vi "parse_variables.vi"(8 "error in (no error)":errorcluster, 9 "Cycles per Experiment":i32=1 min=1 step=1, 10 "Variables (Control)":string[][](table)=[["variable 1", "x", "500", "4000", "1"], ["variable 2", "y", "0", "0", "1"], ["variable 3", "z", "0", "0", "1"], ["", "", "", "", ""], ["", "", "", "", ""], ["", "", "", "", ""], ["", "", "", "", ""], ["", "", "", "", ""]] caption="(Inner loop at top)", 11 "base path":path) -> (0 "error out":errorcluster, 1 "variable indices":i32[][](array[numeric]), 2 "Step Sizes Array":dbl[](array[numeric]), 3 "Variable Names Array":string[](array[string]), 4 "Total Number of Data Points":i32, 5 "variable values":dbl[][](array[numeric]))   [LabVIEW 2013]
doc: "1. Saves off the first column of data as \"plot axis labels\" in \"Processed Data.txt\"\n2. Go through all the possible iterations of the variables, and output a 2D array of those iterations.\n3. Save the data ordering into \"Data Order Log.txt\""
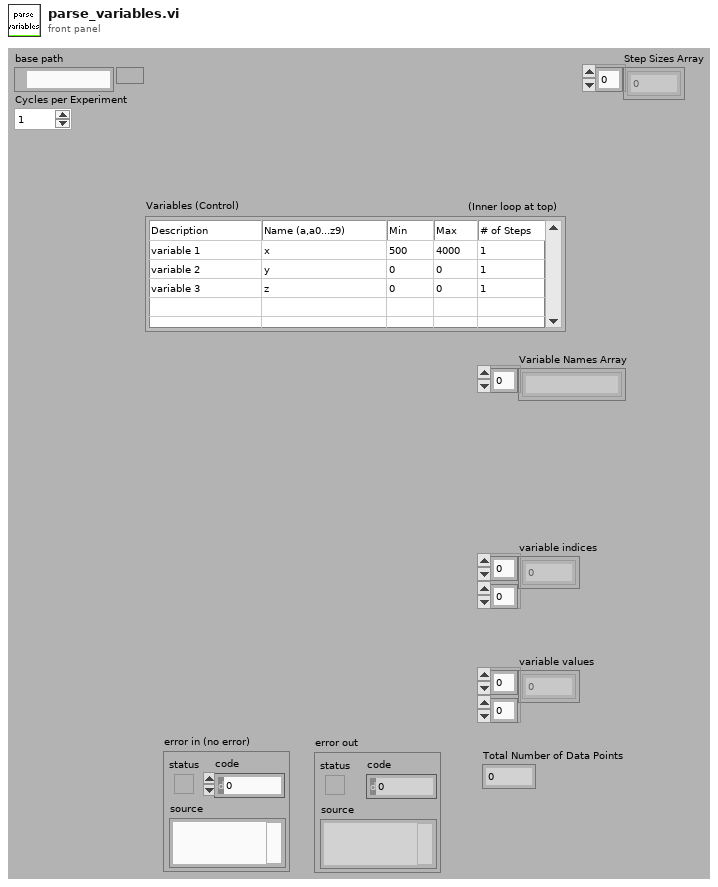
[diagram p1: front panel]
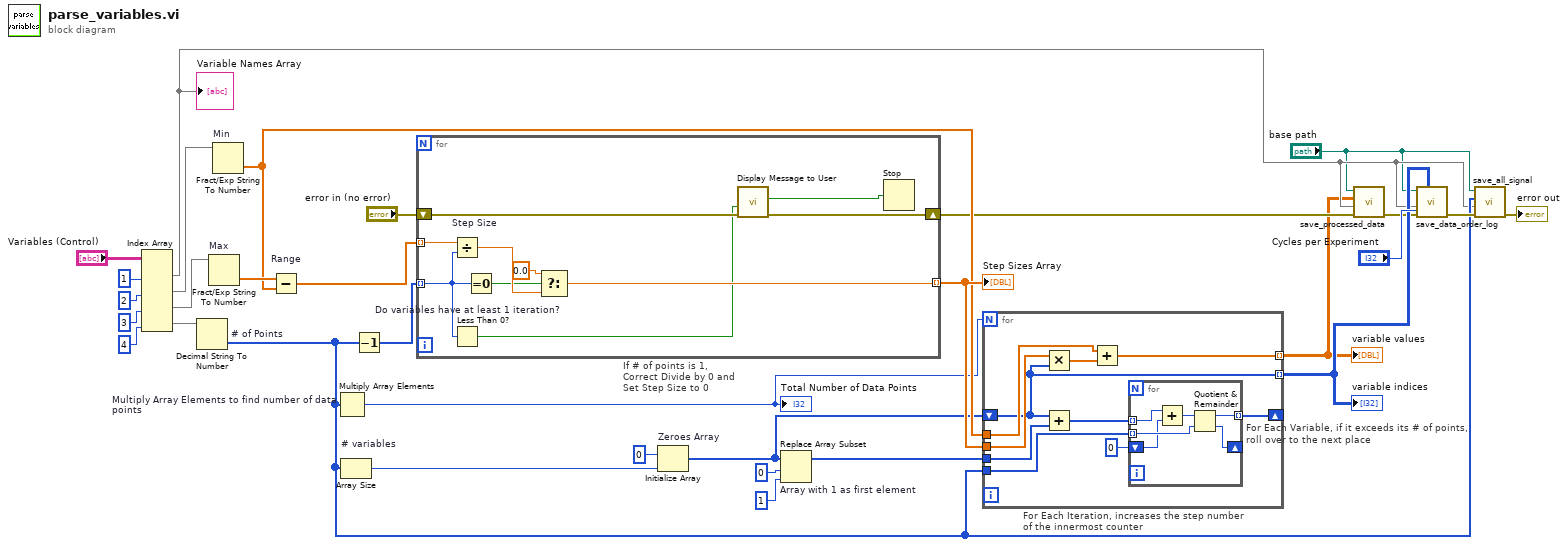
[diagram p0: block diagram]
diagram:
  n1 = Index Array(array="Variables (Control)", index (col) #1=1 ("disabled index (col)"), index (col) #2=2 ("index (col)"), index (col) #3=3 ("index (col)"), index (col) #4=4 ("index (col)")) -> (element #1=w5:string[], element #2=w25:string[], element #3=w24:string[], element #4=w22:string[])  [unwired: 4 in]
  "Variable Names Array" <- w5
  n2 = Decimal String To Number "# of Points"(string=w22) -> (number=w11:i32[])  [unwired: 2 in, 1 out]
  n3 = Fract/Exp String To Number "Max"(string=w24) -> (number=w23:dbl[])  [unwired: 3 in, 1 out]
  n4 = Fract/Exp String To Number "Min"(string=w25) -> (number=w20:dbl[])  [unwired: 3 in, 1 out]
  n5 = Subtract "Range"(x=w23, y=w20) -> (x-y=w30:dbl[])
  n6 = Multiply Array Elements "Multiply Array Elements to find number of data points"(1:w11) -> (0:w16:i32)
  "Total Number of Data Points" <- w16
  n7 = Array Size "# variables"(array=w11) -> (size(s)=w9:i32)
  n8 = Decrement(x=w11) -> (x-1=w31:i32[])
  n9 = for "If # of points is 1, Correct Divide by 0 and Set Step Size to 0" {
    tunnel: [w40] -> w21 mode=indexing
    tunnel: w31 -> [w33] mode=indexing
    tunnel: w30 -> [w39] mode=indexing
    shift-right: [w36] -> w4
    shift-left: "error in (no error)" -> [w35]
    n10 = Divide "Step Size"(x=w39, y=w33) -> (x/y=w38:dbl)
    n11 = Less Than 0? "Do variables have at least 1 iteration?"(x=w33) -> (x < 0?=w32:bool)
    n12 = Equal To 0?(x=w33) -> (x = 0?=w37:bool)
    n13 = Select(t=0.0, s=w37, f=w38) -> (s? t:f=w40:dbl)
    n14 = call "Display Message to User"("error in (no error)"=w35, "Enable"=w32) -> ("error out"=w36:errorcluster, "Stop"=w34:bool)  [unwired: 8 in]
    n15 = Stop(stop? (T)=w34) -> ()
  }
  "Step Sizes Array" <- w21
  n16 = Initialize Array "Zeroes Array"(0, w9) -> (w8:i32[])
  n17 = Replace Array Subset "Array with 1 as first element"(array=w8, new element=1 ("new element/subarray"), index=0) -> (w17:i32[])
  n18 = for "For Each Iteration, increases the step number of the innermost counter" {
    N: w16 -> [_]
    shift-right: [w42] -> _
    shift-left: w8 -> [w43]
    tunnel: w11 -> [w47]
    tunnel: w21 -> [w51]
    tunnel: [w48] -> w1 mode=indexing
    tunnel: w20 -> [w49]
    tunnel: w17 -> [w45]
    tunnel: [w43] -> w12 mode=indexing
    n19 = Multiply(x=w51, y=w43) -> (x*y=w50:dbl[])
    n20 = Add(x=w43, y=w45) -> (x+y=w44:i32[])
    n21 = Add(x=w49, y=w50) -> (x+y=w48:dbl[])
    n22 = for "For Each Variable, if it exceeds its # of points, roll over to the next place" {
      tunnel: w44 -> [w53] mode=indexing
      tunnel: w47 -> [w57] mode=indexing
      shift-right: [w56] -> _
      shift-left: 0 -> [w55]
      tunnel: [w52] -> w42 mode=indexing
      n23 = Add(x=w53, y=w55) -> (x+y=w54:i32)
      n24 = Quotient & Remainder(x=w54, y=w57) -> (x-y*floor(x/y)=w52:i32, floor(x/y)=w56:i32)
    }
  }
  "variable values" <- w1
  "variable indices" <- w12
  n25 = call "save_processed_data.vi"("error in"=w4, "Variable Names Array"=w5, "variable values"=w1, "base path"="base path") -> ("error out"=w3:errorcluster)  [unwired: 7 in]
  n26 = call "save_data_order_log.vi"(6:"Cycles per Experiment", "variable indices"=w12, "error in (no error)"=w3, "Variable Names Array"=w5, "file path"="base path") -> ("error out"=w14:errorcluster)  [unwired: 6 in]
  n27 = call "save_all_signal.vi"("error in (no error)"=w14, "Variable Names Array"=w5, "# of points"=w11, "file path"="base path") -> ("error out"=→"error out":errorcluster)  [unwired: 7 in]
